vi "dispose connection creator.vi"(8 "error in":errorcluster, 11 "conn creator":u64) -> (0 "error out":errorcluster)   [LabVIEW 2016, in "async tls dl.lvlib"]
uses:
  async tls dl.lvlib
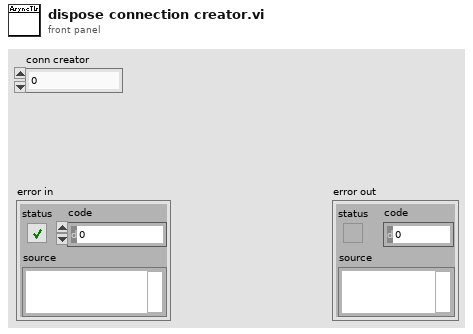
[diagram p1: front panel]
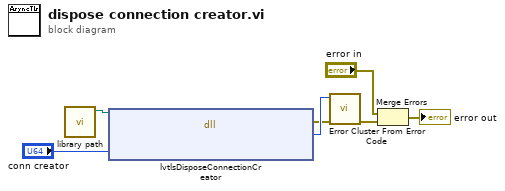
[diagram p0: block diagram]
diagram:
  n1 = call "library path.vi"() -> ("path"=w1:path)  [unwired: 11 in]
  n2 = dll-call lib="C:/Users/IEUser/Desktop/libasynclvtls/lvasynctls.dll" fn="lvtlsDisposeConnectionCreator" ("lvasynctls.dll:lvtlsDisposeClientConnector")(path in=w1, "connCreator"="conn creator") -> (error out=w6:errorcluster, "err"=w7:i32)  [unwired: 3 in, 1 out]
  n3 = call <vilib>:"Error Cluster From Error Code.vi"("error in (no error)"=w6, "error code (0)"=w7) -> ("error out"=w5:errorcluster)  [unwired: 7 in]
  n4 = Merge Errors("error in", w5) -> (→"error out":errorcluster)
